vi "Auto_Routine_StraightTwoPieceTRAJ.vi"(8 "error in (no error)":errorcluster) -> (0 "error out":errorcluster)   [LabVIEW 2023]
doc: "Moves from middle of the speaker to the middle note on robot starting line and back \n*****DOES NOT HAVE WAIT AFTER COMPLETE*****\n-Sets arm to speaker Pose\n-Pre rev\n-Waits for arm (to get to speaker shooot pose)\n-Shoots note\n-Waits for box to shoot note\n-Sets arm to floor\n-Runs intake\n-Moves to note\n-Sets arm to speaker pose\n-20 ms wait\n-Goes back to speaker (while waiting for note to intake and pre rev-ing)\n-Waits for arm (to be at speaker shoot pose)\n-Shoots note\n-Waits for shoot to be done \n-Sets arm to floor"
uses:
  Shoulder/ShoulderGetSetpointEnum.ctl
  Trajectory/TrajectoryGlobals.vi
  <vilib>/Rock Robotics/WPI/ThirdParty/JAS_Junk/TrajLib/Trajectory_Library.lvlib
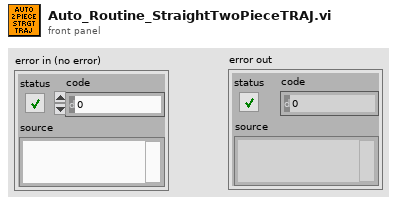
[diagram p1: front panel]
types:
  T1 = typedef "ShoulderGetSetpointEnum.ctl" = enum16{"ShoulderRest", "ShoulderShoot", "ShoulderAmp", "ArmFloorPickup", "ArmAmpDeposit", "ArmSpeakerShoot", "ArmStartPosition", "ArmRestPosition", "ArmSourceIntake", "ArmAwayShoot"}
  T2 = typedef "Trajectory_Library.lvlib/TRAJECTORY.ctl" = cluster{"TotalTImeSecs":dbl, "States":T3[]}
  T3 = typedef "Trajectory_Library.lvlib/TRAJ_STATE.ctl" = cluster{"TimeSeconds":dbl, "Velocity":dbl, "Acceleration":dbl, "POSE":T4, "Curvature":dbl}
  T4 = typedef "Trajectory_Library.lvlib/POSE2D.ctl" = cluster{"TRANSLATION":T5, "ROTATION":T6}
  T5 = typedef "Trajectory_Library.lvlib/TRANSLATION2D.ctl" = cluster{"X":dbl, "Y":dbl}
  T6 = typedef "Trajectory_Library.lvlib/ROTATION2D.ctl" = cluster{"VALUE":dbl, "COS":dbl, "SIN":dbl}
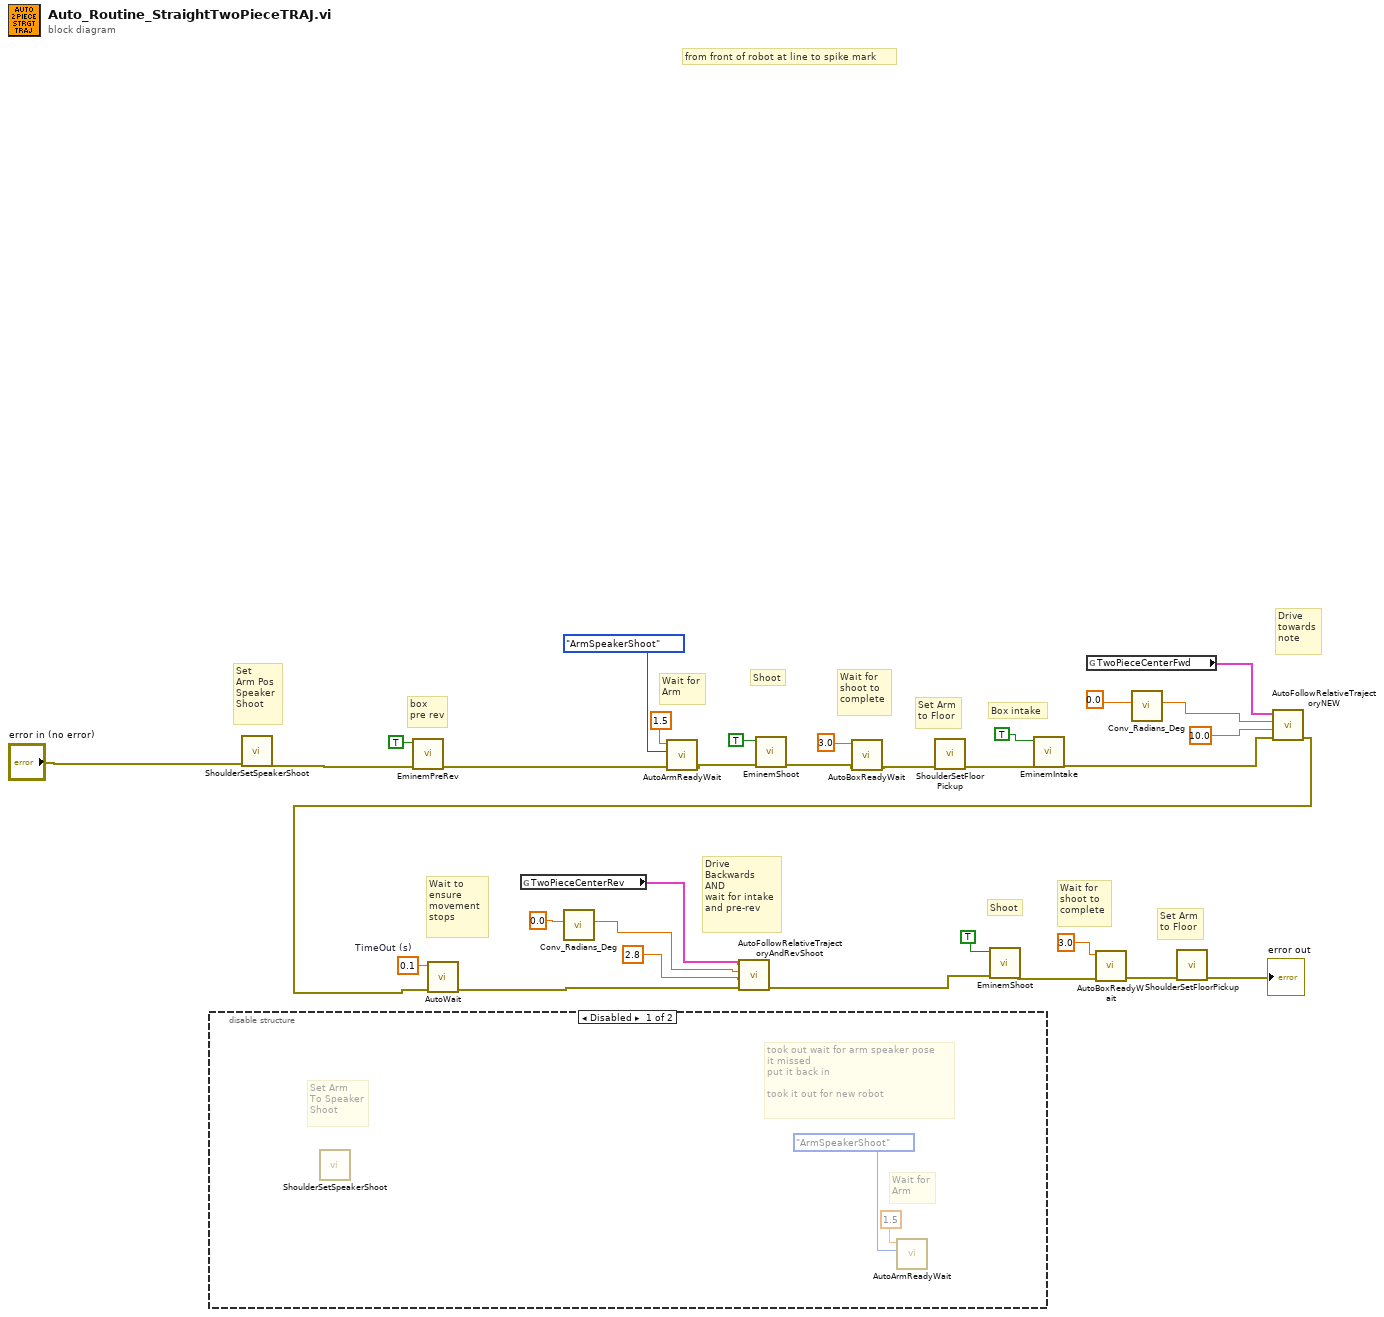
[diagram p0: block diagram]
diagram:
  w5 = 0.1  # TimeOut (s)
  # "Wait to\nensure \nmovement\nstops"
  # "Set Arm\nto Floor"
  # "Wait for\nshoot to\ncomplete"
  # "Shoot"
  # "Drive\nBackwards\nAND\nwait for intake\nand pre-rev"
  # "Drive\ntowards\nnote"
  # "box \npre rev"
  # "Box intake"
  # "Set Arm\nto Floor"
  # "Wait for\nshoot to\ncomplete"
  # "Shoot"
  # "Wait for\nArm"
  # "Set\nArm Pos\nSpeaker\nShoot"
  # "from front of robot at line to spike mark"
  n1 = disable-structure shown="Disabled" {
    frame Disabled {
      # "Wait for\nArm"
      # "took out wait for arm speaker pose \nit missed\nput it back in\n\ntook it out for new robot"
      # "Set Arm\nTo Speaker\nShoot"
      n2 = call "ShoulderSetSpeakerShoot.vi"() -> ()  [unwired: 11 in, 1 out]
      n3 = call "AutoArmReadyWait.vi"("ArmSetpoints"=ShoulderGetSetpointEnum."ArmSpeakerShoot", "TimeOut (s)"=1.5) -> ("error in (no error)"=w32:errorcluster)  [unwired: 8 in, 1 out]
    }
    frame Enabled {
    }
  }
  n4 = call "ShoulderSetSpeakerShoot.vi"("error in (no error)"="error in (no error)") -> ("error out"=w15:errorcluster)  [unwired: 10 in]
  n5 = call "EminemPreRev.vi"("error in"=w15, "PreRev"=TRUE) -> ("error out"=w17:errorcluster)  [unwired: 9 in]
  n6 = global read "TrajectoryGlobals.vi" "TwoPieceCenterRev"() -> (w9:T2)
  n7 = call <vilib>:"Conv_Radians_Deg.vi"("Radians"=0.0) -> ("Degrees"=w8:dbl)  [unwired: 10 in]
  n8 = call "AutoArmReadyWait.vi"("error in (no error)"=w17, "ArmSetpoints"=ShoulderGetSetpointEnum."ArmSpeakerShoot", "TimeOut (s)"=1.5) -> ("error out"=w26:errorcluster)  [unwired: 8 in]
  n9 = call "EminemShoot.vi"("error in (no error)"=w26, "Box shoot"=TRUE) -> ("error out"=w28:errorcluster)  [unwired: 9 in]
  n10 = call "AutoBoxReadyWait.vi"("error in (no error)"=w28, "TimeOut (s)"=3.0) -> ("error out"=w29:errorcluster)  [unwired: 9 in]
  n11 = call "ShoulderSetFloorPickup.vi"("error in (no error)"=w29) -> ("error out"=w25:errorcluster)  [unwired: 10 in]
  n12 = call "EminemIntake.vi"("error in (no error)"=w25, "Box intake"=TRUE) -> ("error out"=w18:errorcluster)  [unwired: 9 in]
  n13 = global read "TrajectoryGlobals.vi" "TwoPieceCenterFwd"() -> (w22:T2)
  n14 = call <vilib>:"Conv_Radians_Deg.vi"("Radians"=0.0) -> ("Degrees"=w20:dbl)  [unwired: 10 in]
  n15 = call "AutoFollowRelativeTrajectoryNEW.vi"("error in (no error)"=w18, "TimeOut (s)"=10.0, "End Orientation"=w20, "Trajectory"=w22) -> ("error out"=w2:errorcluster)  [unwired: 7 in]
  n16 = call "AutoWait.vi"("error in (no error)"=w2, "TimeOut (s)"=w5) -> ("error out"=w6:errorcluster)  [unwired: 9 in]
  n17 = call "AutoFollowRelativeTrajectoryAndRevShoot.vi"("error in (no error)"=w6, "TimeOut (s)"=2.8, "End Orientation"=w8, "Trajectory"=w9) -> ("error out"=w1:errorcluster)  [unwired: 7 in]
  n18 = call "EminemShoot.vi"("error in (no error)"=w1, "Box shoot"=TRUE) -> ("error out"=w13:errorcluster)  [unwired: 9 in]
  n19 = call "AutoBoxReadyWait.vi"("error in (no error)"=w13, "TimeOut (s)"=3.0) -> ("error out"=w10:errorcluster)  [unwired: 9 in]
  n20 = call "ShoulderSetFloorPickup.vi"("error in (no error)"=w10) -> ("error out"=→"error out":errorcluster)  [unwired: 10 in]
